vi "dfd_Halfband Filter Design Lowpass to Highpass.vi"(8 "error in (no error)":errorcluster, 10 "filter type":enum16{"Lowpass", "Highpass"}(ring), 11 "h in":dbl[](array[numeric])) -> (0 "error out":errorcluster, 3 "h out":dbl[](array[numeric]))   [LabVIEW 2017, in "NI_DigFilter_Process.lvlib"]
uses:
  <vilib>/addons/Digital Filter Design/NI_DigFilter_Process.lvlib
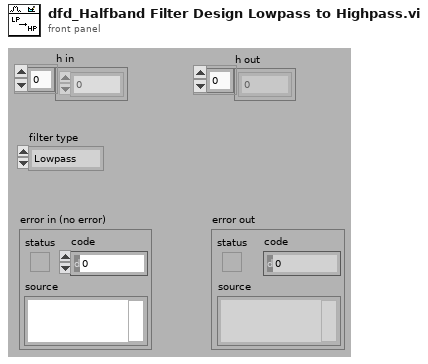
[diagram p1: front panel]
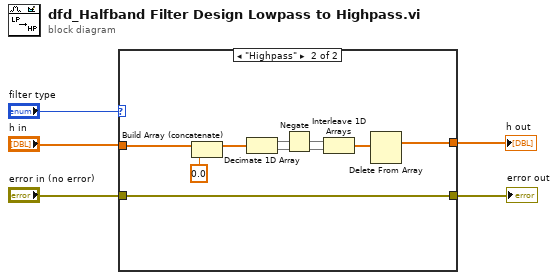
[diagram p0: block diagram]
diagram:
  n1 = case shown="\"Highpass\"" "filter type" {
    tunnel: "h in" -> [w7 w10]
    tunnel: [w7 w9] -> w3
    tunnel: [w6 w8] -> w1
    tunnel: "error in (no error)" -> [w6 w8]
    frame "Lowpass", Default {
    }
    frame "Highpass" {
      n2 = Build Array (concatenate)(w10, 0.0) -> (w15:dbl[])
      n3 = Decimate 1D Array(w15) -> (w13:dbl[], w12:dbl[])
      n4 = Negate(x=w13) -> (-x=w11:dbl[])
      n5 = Interleave 1D Arrays(w11, w12) -> (w14:dbl[])
      n6 = Delete From Array(array=w14) -> (array with subset deleted=w9:dbl[])  [unwired: 2 in, 1 out]
    }
  }
  "h out" <- w3
  "error out" <- w1
